vi "Configure Grating.vi"(7 "turret index (0)":u8, 8 "error in (no error)":errorcluster, 10 "grating index":u8, 11 "SOL MS in":refnum<class "PL SOL Instruments MS.lvclass">) -> (0 "error out":errorcluster, 1 "dispersion, nm/mm":dbl, 2 "wavelength, nm":dbl, 3 "SOL MS out":refnum<class "PL SOL Instruments MS.lvclass">)   [LabVIEW 2015, in "PL SOL Instruments MS.lvclass"]
doc: "Configures grating."
uses:
  PL SOL Instruments MS.lvclass
  PL SOL Instruments MS.lvclass/PL SOL Instruments MS.ctl
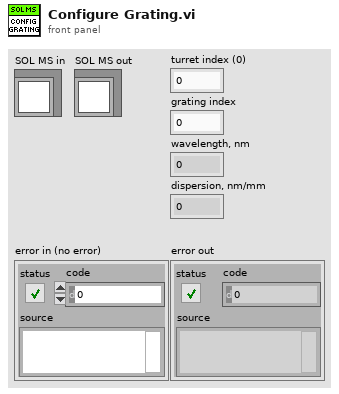
[diagram p1: front panel]
types:
  T1 = cluster{"name":string, "step timeout, ms":u32, "reset timeout, ms":u32, "gratings":cluster{"name":string, "step timeout, ms":u32, "reset timeout, ms":u32, "turret position":i32, "reset position":i32, "max position":i32, "backlash distance":i32, "step size, rad":dbl, "groove density, g/mm":dbl, "theta2, rad":dbl, "blaze wavelength, nm":dbl, "focal length, cm":dbl, "manual change":bool, "manual change position":i32}[], "current grating":cluster{"index":u8, "position":i32}}[]
  T2 = cluster{"name":string, "step timeout, ms":u32, "reset timeout, ms":u32, "gratings":cluster{"name":string, "step timeout, ms":u32, "reset timeout, ms":u32, "turret position":i32, "reset position":i32, "max position":i32, "backlash distance":i32, "step size, rad":dbl, "groove density, g/mm":dbl, "theta2, rad":dbl, "blaze wavelength, nm":dbl, "focal length, cm":dbl, "manual change":bool, "manual change position":i32}[], "current grating":cluster{"index":u8, "position":i32}}
  T3 = cluster{"name":string, "step timeout, ms":u32, "reset timeout, ms":u32, "turret position":i32, "reset position":i32, "max position":i32, "backlash distance":i32, "step size, rad":dbl, "groove density, g/mm":dbl, "theta2, rad":dbl, "blaze wavelength, nm":dbl, "focal length, cm":dbl, "manual change":bool, "manual change position":i32}[]
  T4 = cluster{"turrets":cluster{"current grating index":u8, "wavelength, nm":dbl, "dispersion, nm/mm":dbl}[], "shutters":cluster{"is open":bool}[], "mirrors":cluster{"current position index":u8}[], "slits":cluster{"width, um":dbl}[]}
  T5 = cluster{"name":string, "step timeout, ms":u32, "reset timeout, ms":u32, "turret position":i32, "reset position":i32, "max position":i32, "backlash distance":i32, "step size, rad":dbl, "groove density, g/mm":dbl, "theta2, rad":dbl, "blaze wavelength, nm":dbl, "focal length, cm":dbl, "manual change":bool, "manual change position":i32}
  T6 = cluster{"current grating index":u8, "wavelength, nm":dbl, "dispersion, nm/mm":dbl}[]
  T7 = cluster{"current grating index":u8, "wavelength, nm":dbl, "dispersion, nm/mm":dbl}
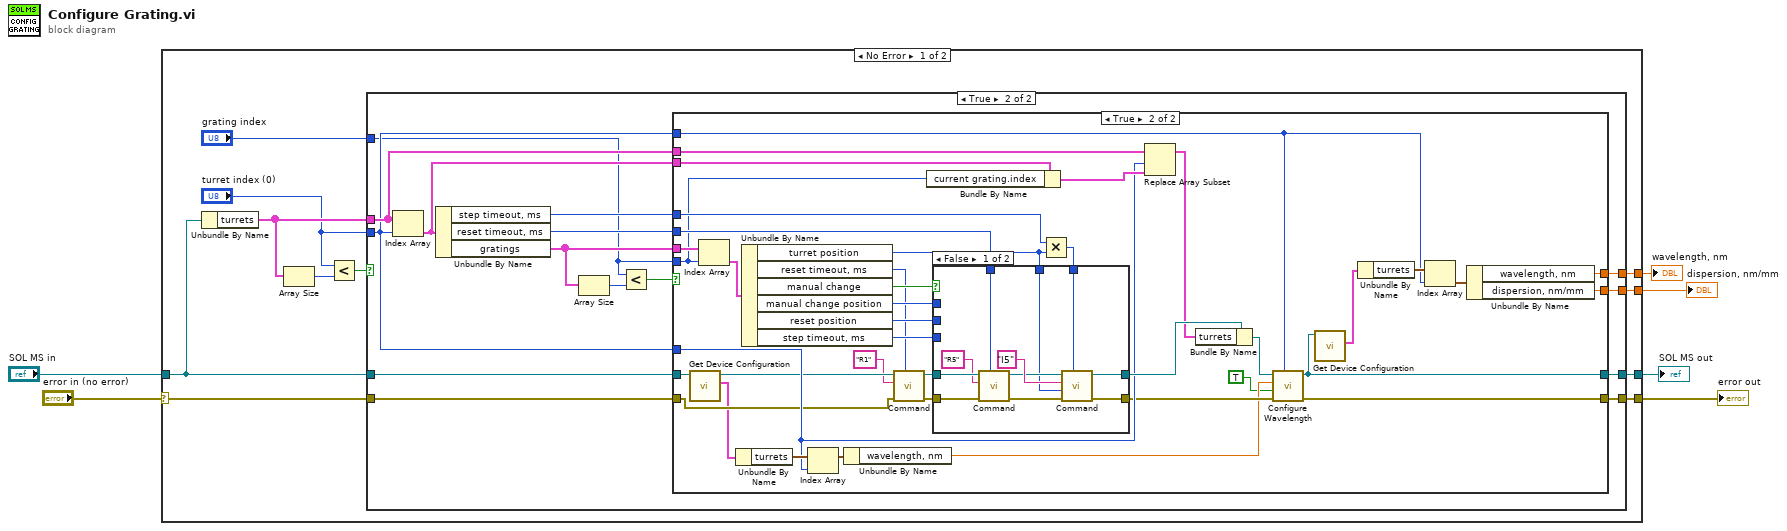
[diagram p0: block diagram]
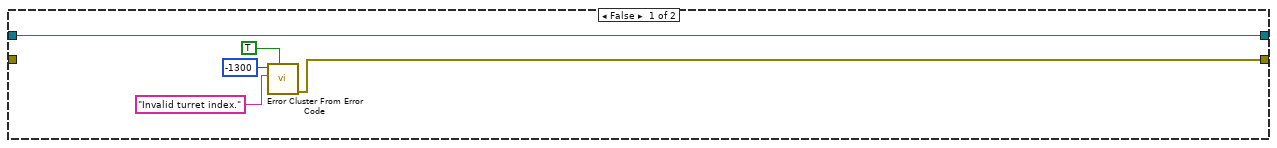
[diagram p2: hidden frame]
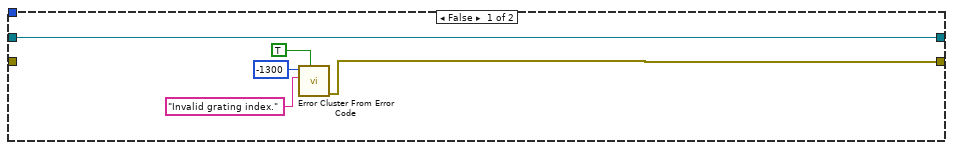
[diagram p3: hidden frame]
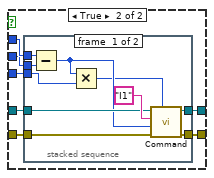
[diagram p4: hidden frame]
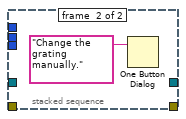
[diagram p5: hidden frame]
diagram:
  n1 = case shown="No Error" "error in (no error)" {
    selector: "error in (no error)" -> [w11 w111]
    tunnel: "SOL MS in" -> [w17 w112]
    tunnel: [w10 w112] -> w5
    tunnel: [w9 w111] -> w4
    tunnel: [w8 _] -> w3
    tunnel: [w7 _] -> w2
    frame No Error {
      n2 = Unbundle By Name(w17) -> ("turrets"=w16:T1)
      n3 = Array Size(array=w16) -> (size(s)=w14:i32)
      n4 = Less?(x="turret index (0)", y=w14) -> (x < y?=w13:bool)
      n5 = case shown="True" w13 {
        tunnel: w11 -> [_ w29]
        tunnel: w17 -> [w22 w30]
        tunnel: [w22 w37] -> w10
        tunnel: [w21 w36] -> w9
        tunnel: w16 -> [_ w32]
        tunnel: "grating index" -> [_ w23]
        tunnel: "turret index (0)" -> [_ w27]
        tunnel: [_ w26] -> w8
        tunnel: [_ w25] -> w7
        frame False {
          n6 = call <vilib>:"Error Cluster From Error Code.vi"("show call chain? (False)"=TRUE, "error message (\"\")"="Invalid turret index." ("error message (\"\")"), "error code (0)"=-1300) -> ("error out"=w21:errorcluster)  [unwired: 6 in]
        }
        frame True {
          n7 = Index Array(array=w32, index=w27) -> (element=w31:T2)
          n8 = Unbundle By Name(w31) -> ("step timeout, ms"=w33:u32, "reset timeout, ms"=w34:u32, "gratings"=w35:T3)
          n9 = Array Size(array=w35) -> (size(s)=w24:i32)
          n10 = Less?(x=w23, y=w24) -> (x < y?=w28:bool)
          n11 = case shown="True" w28 {
            tunnel: w29 -> [_ w58]
            tunnel: w30 -> [w42 w62]
            tunnel: [w42 w46] -> w37
            tunnel: [w41 w54] -> w36
            tunnel: w35 -> [_ w81]
            tunnel: w23 -> [_ w74]
            tunnel: w34 -> [_ w79]
            tunnel: w33 -> [_ w77]
            tunnel: w27 -> [_ w66]
            tunnel: w32 -> [_ w75]
            tunnel: w31 -> [_ w68]
            tunnel: w27 -> [_ w45]
            tunnel: [_ w44] -> w26
            tunnel: [_ w43] -> w25
            frame False {
              n12 = call <vilib>:"Error Cluster From Error Code.vi"("show call chain? (False)"=TRUE, "error message (\"\")"="Invalid grating index." ("error message (\"\")"), "error code (0)"=-1300) -> ("error out"=w41:errorcluster)  [unwired: 6 in]
            }
            frame True {
              n13 = call "Get Device Configuration.vi"("SOL MS in"=w62) -> ("configuration"=w55:T4, "SOL MS out"=w61:refnum<class "PL SOL Instruments MS.lvclass">)  [unwired: 9 in]
              n14 = Index Array(array=w81, index=w74) -> (element=w80:T5)
              n15 = Unbundle By Name(w55) -> ("turrets"=w69:T6)
              n16 = Unbundle By Name(w80) -> ("turret position"=w78:i32, "reset timeout, ms"=w59:u32, "manual change"=w67:bool, "manual change position"=w65:i32, "reset position"=w64:i32, "step timeout, ms"=w63:u32)
              n17 = Index Array(array=w69, index=w66) -> (element=w70:T7)
              n18 = Unbundle By Name(w70) -> ("wavelength, nm"=w51:dbl)
              n19 = call "Command.vi"("additional timeout, ms (0)"=w59, "error in (no error)"=w58, "command"="R1", "SOL MS in"=w61) -> ("error out"=w57:errorcluster, "SOL MS out"=w56:refnum<class "PL SOL Instruments MS.lvclass">)  [unwired: 6 in]
              n20 = Bundle By Name(cluster=w68, "current grating.index"=w74) -> (w73:T2)
              n21 = Multiply(x=w77, y=w78) -> (x*y=w76:u32)
              n22 = case shown="False" w67 {
                tunnel: w79 -> [w91 _]
                tunnel: w78 -> [w83 _]
                tunnel: w76 -> [w87 _]
                tunnel: [w86 w96] -> w53
                tunnel: [w88 w97] -> w72
                tunnel: w56 -> [w92 w99]
                tunnel: w57 -> [w90 w98]
                tunnel: w65 -> [_ w95]
                tunnel: w64 -> [_ w94]
                tunnel: w63 -> [_ w93]
                frame False {
                  n23 = call "Command.vi"("additional timeout, ms (0)"=w91, "error in (no error)"=w90, "command"="R5", "SOL MS in"=w92) -> ("error out"=w82:errorcluster, "SOL MS out"=w84:refnum<class "PL SOL Instruments MS.lvclass">)  [unwired: 6 in]
                  n24 = call "Command.vi"("additional timeout, ms (0)"=w87, "error in (no error)"=w82, "data"=w83, "command"="I5", "SOL MS in"=w84) -> ("error out"=w86:errorcluster, "SOL MS out"=w88:refnum<class "PL SOL Instruments MS.lvclass">)  [unwired: 5 in]
                }
                frame True {
                  n25 = stacked-sequence {
                    tunnel: w99 -> [w104 _]
                    tunnel: w98 -> [w103 _]
                    tunnel: [w105 _] -> w97
                    tunnel: [w102 _] -> w96
                    tunnel: w95 -> [w109 _]
                    tunnel: w94 -> [w108 _]
                    tunnel: w93 -> [w107 _]
                    frame #0 {
                      n26 = Subtract(x=w109, y=w108) -> (x-y=w101:i32)
                      n27 = Multiply(x=w101, y=w107) -> (x*y=w100:u32)
                      n28 = call "Command.vi"("additional timeout, ms (0)"=w100, "error in (no error)"=w103, "data"=w101, "command"="I1", "SOL MS in"=w104) -> ("error out"=w102:errorcluster, "SOL MS out"=w105:refnum<class "PL SOL Instruments MS.lvclass">)  [unwired: 5 in]
                    }
                    frame #1 {
                      n29 = One Button Dialog(message="Change the grating manually.") -> ()  [unwired: 1 in, 1 out]
                    }
                  }
                }
              }
              n30 = Replace Array Subset(array=w75, new element=w73, index=w66) -> (w71:T1)
              n31 = Bundle By Name(cluster=w72, "turrets"=w71) -> (w52:refnum<class "PL SOL Instruments MS.lvclass">)
              n32 = call "Configure Wavelength.vi"("turret index (0)"=w45, "error in (no error)"=w53, "reset (false)"=TRUE ("reset"), "wavelength, nm"=w51, "SOL MS in"=w52) -> ("error out"=w54:errorcluster, "SOL MS out"=w46:refnum<class "PL SOL Instruments MS.lvclass">)  [unwired: 3 in, 2 out]
              n33 = call "Get Device Configuration.vi"("SOL MS in"=w46) -> ("configuration"=w47:T4)  [unwired: 9 in, 1 out]
              n34 = Unbundle By Name(w47) -> ("turrets"=w49:T6)
              n35 = Index Array(array=w49, index=w45) -> (element=w48:T7)
              n36 = Unbundle By Name(w48) -> ("wavelength, nm"=w44:dbl, "dispersion, nm/mm"=w43:dbl)
            }
          }
        }
      }
    }
    frame Error {
    }
  }
  "SOL MS out" <- w5
  "wavelength, nm" <- w3
  "dispersion, nm/mm" <- w2
  "error out" <- w4
